vi "FM_RTL-SDR_RX-COM.vi"() -> ()   [LabVIEW 2013]
uses:
  <vilib>/sound2/lvsound2.llb/Sound Data Format.ctl
  <vilib>/sound2/lvsound2.llb/Sound Output Write (DBL Single).vi
  <vilib>/Analysis/2dsp.llb/Rational Resample (single channel, DBL).vi
  <instrlib>/rtlsdr/rtlsdrx64.lvlib
  <vilib>/Analysis/NI_AALPro.lvlib
panel:
  out "Boolean":bool
  out "error out":errorcluster
  out "error out":errorcluster
  in  "Device index":u32
  out "Samples Acquired":u32
  out "DevRefnum":u64
  out "error out":errorcluster
  in  "sound format":T1={"sample rate (S/s)"=44100.0, "number of channels"=1, "bits per sample"=16}
  in  "stop":bool
  in  "中心频率：":u32(slide)=104300000 scale=86000000.0..108000000.0 scale format="%#_6p"
  in  "IQ rate":u32=286650
  out "error out":errorcluster
  # "FM Receiver"
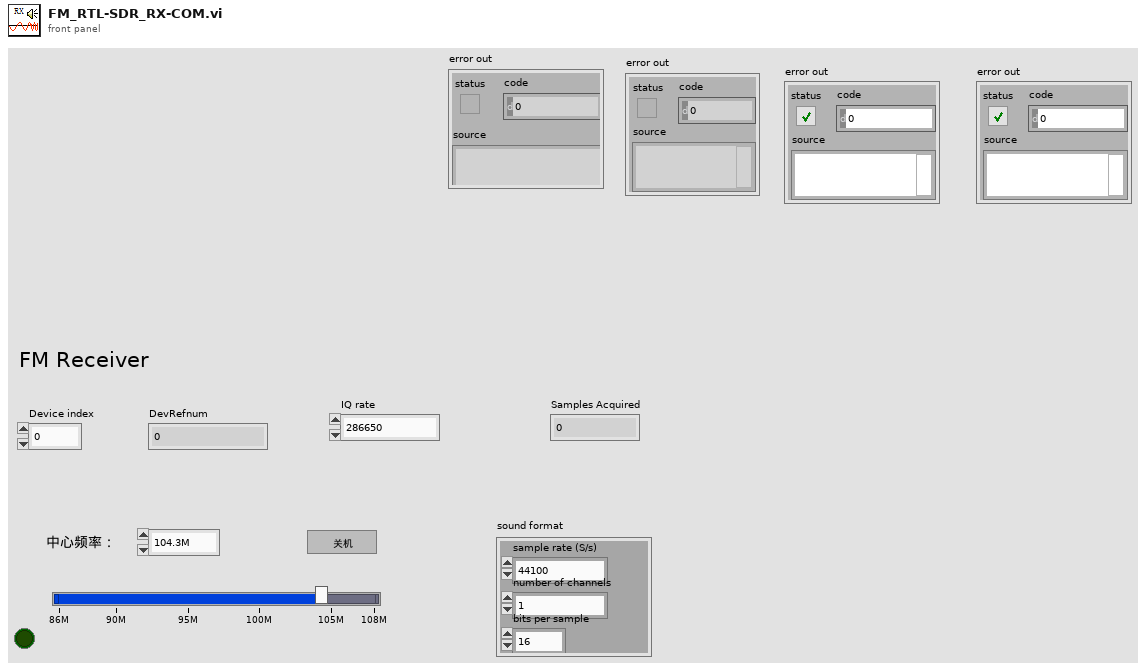
[diagram p1: front panel]
types:
  T1 = typedef "Sound Data Format.ctl" = cluster{"sample rate (S/s)":dbl, "number of channels":i32, "bits per sample":i32}
  T2 = typedef "Sound Output Task ID.ctl" = u32
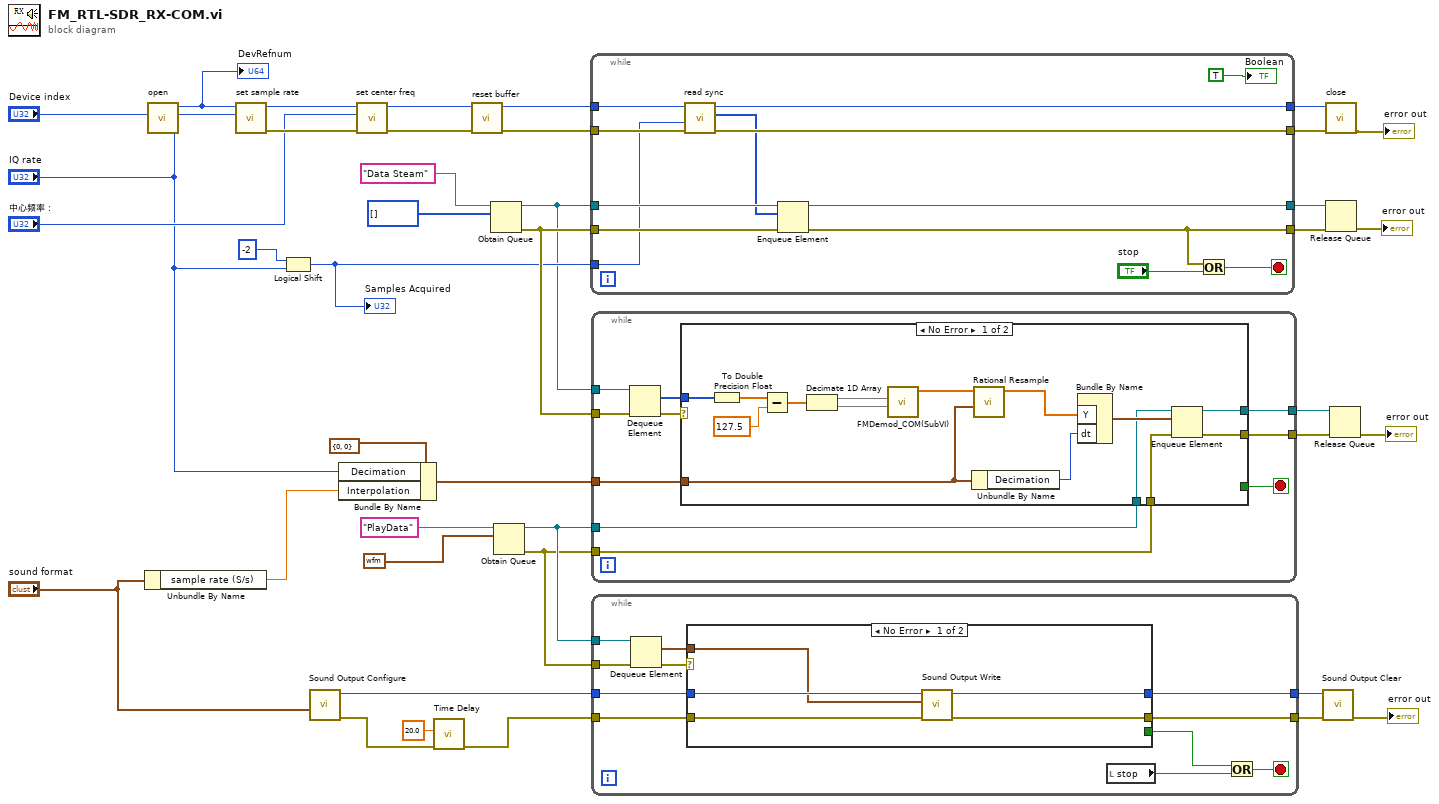
[diagram p0: block diagram]
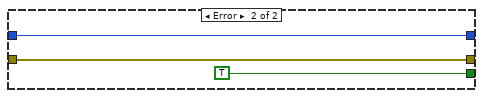
[diagram p2: hidden frame]
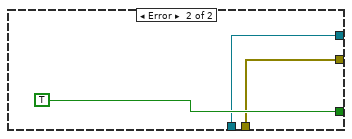
[diagram p3: hidden frame]
diagram:
  n1 = Unbundle By Name("sound format") -> ("sample rate (S/s)"=w13:dbl)
  n2 = call <instrlib>:"open.vi"("index"="Device index") -> ("DevRefnum"=w33:u64)  [unwired: 9 in, 1 out]
  "DevRefnum" <- w33
  n3 = call <instrlib>:"set sample rate.vi"("rate"="IQ rate", "DevRefnum"=w33) -> ("error out"=w35:errorcluster, "DevRefnum"=w37:u64)  [unwired: 7 in, 1 out]
  n4 = Logical Shift(y=i16 -2, x="IQ rate") -> (x << y=w16:u32)
  "Samples Acquired" <- w16
  n5 = call <vilib>:"Sound Output Configure.vi"("sound format"="sound format") -> ("error out"=w20:errorcluster, "task ID"=w10:T2)  [unwired: 9 in]
  n6 = Bundle By Name(cluster=cluster{"Interpolation":i32, "Decimation":i32} {"Interpolation"=0, "Decimation"=0}, "Decimation"="IQ rate", "Interpolation"=w13) -> (w21:cluster{"Interpolation":i32, "Decimation":i32})
  n7 = call <instrlib>:"set center freq.vi"("error in (no error)"=w35, "freq"="中心频率：", "DevRefnum"=w37) -> ("error out"=w34:errorcluster, "DevRefnum"=w36:u64)  [unwired: 6 in, 1 out]
  n8 = call "Time Delay"("error in (no error)"=w20, "Delay Time (s)"=20.0) -> ("error out"=w7:errorcluster)  [unwired: 9 in]
  n9 = call <instrlib>:"reset buffer.vi"("error in (no error)"=w34, "DevRefnum"=w36) -> ("error out"=w30:errorcluster, "DevRefnum"=w31:u64)  [unwired: 8 in]
  n10 = Obtain Queue(name (unnamed)="Data Steam", element data type=u8[] [] ("buf 2")) -> (queue out=w15:refnum<queue>, error out=w17:errorcluster)  [unwired: 3 in, 1 out]
  n11 = Obtain Queue(name (unnamed)="PlayData", element data type=waveform(dbl) {"t0"=timestamp(0 s since 1904-01-01), "dt"=1.0, "Y"=[]} ("waveform")) -> (queue out=w8:refnum<queue>, error out=w4:errorcluster)  [unwired: 3 in, 1 out]
  n12 = while {
    tunnel: [w51] -> w28
    tunnel: w31 -> [w53]
    tunnel: w30 -> [w52]
    tunnel: [w50] -> w27
    tunnel: w16 -> [w42]
    tunnel: w15 -> [w49]
    tunnel: [w48] -> w24
    tunnel: w17 -> [w47]
    tunnel: [w45] -> w23
    stop <- w43 stop-if-true
    n13 = call <instrlib>:"read sync.vi"("error in (no error)"=w52, "len"=w42, "DevRefnum"=w53) -> ("error out"=w50:errorcluster, "buf 2"=w46:u8[], "DevRefnum"=w51:u64)  [unwired: 6 in]
    n14 = Enqueue Element(queue=w49, element=w46, error in (no error)=w47) -> (queue out=w48:refnum<queue>, error out=w45:errorcluster)  [unwired: 1 in, 1 out]
    n15 = Or(x=w45, y="stop") -> (x .or. y?=w43:bool)
    "Boolean" <- TRUE
  }
  n16 = while {
    tunnel: w15 -> [w63]
    tunnel: w21 -> [w58]
    tunnel: w17 -> [w61]
    tunnel: w8 -> [w57]
    tunnel: w4 -> [w56]
    tunnel: [w55] -> w2
    tunnel: [w54] -> w1
    stop <- w59 stop-if-true
    n17 = Dequeue Element(queue=w63, error in (no error)=w61) -> (element=w62:u8[], error out=w60:errorcluster)  [unwired: 1 in, 2 out]
    n18 = case shown="No Error" w60 {
      tunnel: w62 -> [w75 _]
      tunnel: [_ TRUE] -> w59
      tunnel: w58 -> [w72 _]
      tunnel: w57 -> [w70 w80]
      tunnel: w56 -> [w69 w79]
      tunnel: [w68 w80] -> w55
      tunnel: [w67 w79] -> w54
      frame No Error {
        n19 = To Double Precision Float(number=w75) -> (double precision float=w78:dbl[])
        n20 = Subtract(x=w78, y=127.5) -> (x-y=w76:dbl[])
        n21 = Decimate 1D Array(w76) -> (w66:dbl[], w65:dbl[])
        n22 = call "FMDemod_COM(SubVI).vi"("QSamples"=w65, "ISamples"=w66) -> ("Baseband"=w64:dbl[])  [unwired: 9 in]
        n23 = Unbundle By Name(w72) -> ("Decimation"=w73:i32)
        n24 = call-poly <vilib>:"Rational Resample.vi"("resample factor"=w72, "X"=w64) -> ("Y"=w74:dbl[])  [unwired: 7 in, 2 out]
        n25 = Bundle By Name ("Build Waveform")("Y"=w74, "dt"=w73) -> (w71:waveform(dbl))  [unwired: 1 in]
        n26 = Enqueue Element(queue=w70, element=w71, error in (no error)=w69) -> (queue out=w68:refnum<queue>, error out=w67:errorcluster)  [unwired: 1 in, 1 out]
      }
      frame Error {
      }
    }
  }
  n27 = while {
    tunnel: w10 -> [w92]
    tunnel: [w91] -> w9
    tunnel: w8 -> [w90]
    tunnel: w4 -> [w89]
    tunnel: w7 -> [w88]
    tunnel: [w87] -> w6
    stop <- w82 stop-if-true
    n28 = Dequeue Element(queue=w90, error in (no error)=w89) -> (element=w85:waveform(dbl), error out=w86:errorcluster)  [unwired: 1 in, 2 out]
    n29 = case shown="No Error" w86 {
      tunnel: w92 -> [w97 w100]
      tunnel: [w96 w100] -> w91
      tunnel: w88 -> [w95 w99]
      tunnel: [w94 w99] -> w87
      tunnel: w85 -> [w93 _]
      tunnel: [_ TRUE] -> w84
      frame No Error {
        n30 = call-poly <vilib>:"Sound Output Write.vi"("error in (no error)"=w95, "data"=w93, "task ID"=w97) -> ("error out"=w94:errorcluster, "task ID out"=w96:T2)  [unwired: 7 in]
      }
      frame Error {
      }
    }
    n31 = local read "stop"() -> (w83:bool)
    n32 = Or(x=w84, y=w83) -> (x .or. y?=w82:bool)
  }
  n33 = call <vilib>:"Sound Output Clear.vi"("error in (no error)"=w6, "task ID"=w9) -> ("error out"=→"error out":errorcluster)  [unwired: 9 in]
  n34 = call <instrlib>:"close.vi"("error in (no error)"=w27, "DevRefnum"=w28) -> ("error out"=→"error out":errorcluster)  [unwired: 8 in, 1 out]
  n35 = Release Queue(queue=w24, error in (no error)=w23) -> (error out=→"error out":errorcluster)  [unwired: 1 in, 2 out]
  n36 = Release Queue(queue=w2, error in (no error)=w1) -> (error out=→"error out":errorcluster)  [unwired: 1 in, 2 out]
